vi "Get Valid Item Ref.vi"(8 "error in (no error)":errorcluster, 9 "scalar channels":T1 {"Data Type" format="%.0x"}, 10 "bitfile object names":string[](array[string]), 11 "section children refs":T3[](array[typedef]) format="%.0x") -> (0 "error out":errorcluster, 1 "scalar channel out":T1 {"Data Type" format="%.0x"}, 2 "Not a Ref":bool, 3 "item ref out":T3 format="%.0x")   [LabVIEW 2018, in "FPGA Addon System Explorer.lvlib"]
uses:
  FPGA Addon System Explorer.lvlib
  Addon Shared/Types/Register Information.ctl
  Addon Shared/Types/Data Type.ctl
  <vilib>/NI Veristand/Custom Device API/Custom Device Item Ref.ctl
  <vilib>/NI Veristand/Custom Device Tools/Custom Device Utility Library/Custom Device Utility Library.lvlib
  <vilib>/NI Veristand/Custom Device API/Custom Device API.lvlib
  Addon Shared/FPGA Addon Shared.lvlib
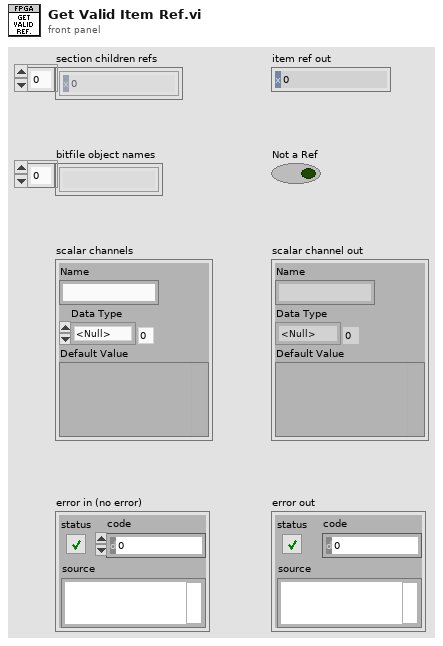
[diagram p1: front panel]
types:
  T1 = typedef "FPGA Addon Shared.lvlib/Register Information.ctl" = cluster{"Name":string, "Data Type":T2, "Default Value":variant}
  T2 = typedef "FPGA Addon Shared.lvlib/Data Type.ctl" = enum8{"<Null>", "I8", "I16", "I32", "I64", "U8", "U16", "U32", "U64", "SGL", "Boolean", "Analog PWM In Settings", "Analog PWM In", "Digital PWM In Settings", "Digital PWM In", "Digital PWM Out", "Sine Out", "FXP+/-24.5", "FXP+/-16.5", "FXP+/-32.8", "FXP+/-64.32", "FXP+/-16.7", "FXP+/-20.5", "FXP+/-27.5", "FXP+/-32.16", "FXP+16.3", "FXP+18.3", "Digital Static In", "Digital Static Out", "Digital Static In Settings", "Digital WSS Out", "Quad Encoder Settings", "Quad Encoder In", "Group"}
  T3 = typedef "Custom Device API.lvlib/Custom Device Item Ref.ctl" = u64
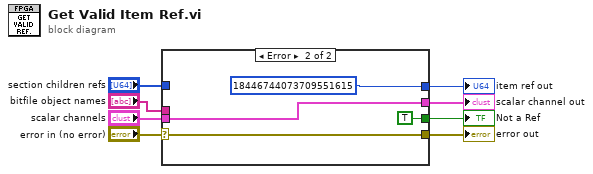
[diagram p0: block diagram]
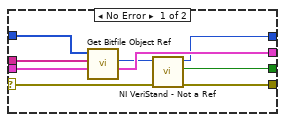
[diagram p2: hidden frame]
diagram:
  n1 = case shown="Error" "error in (no error)" {
    selector: "error in (no error)" -> [w9 w21]
    tunnel: [w17 w20] -> w8
    tunnel: [w16 T3 18446744073709551615 ("Scalar Section ref")] -> w7
    tunnel: [w15 TRUE ("Not a Ref")] -> w6
    tunnel: [w13 w21] -> w5
    tunnel: "section children refs" -> [w12 _]
    tunnel: "scalar channels" -> [w11 w20]
    tunnel: "bitfile object names" -> [w10 _]
    frame No Error {
      n2 = call "Get Bitfile Object Ref.vi"("scalar channel in"=w11, "bitfile object names"=w10, "section children refs in"=w12) -> ("scalar channel out"=w17:T1, "item ref out"=w14:T3)  [unwired: 6 in, 1 out]
      n3 = call <vilib>:"NI VeriStand - Not a Ref.vi"("error in (no error)"=w9, "Item Ref"=w14) -> ("error out"=w13:errorcluster, "Not a Ref"=w15:bool, "Item Ref out"=w16:T3)  [unwired: 7 in]
    }
    frame Error {
    }
  }
  "scalar channel out" <- w8
  "item ref out" <- w7
  "Not a Ref" <- w6
  "error out" <- w5
